vi "brc_daq_get_last_error.vi"(0 "return_value":i32) -> (19 "error out":errorcluster)   [LabVIEW 2019, in "BRC-DAQ.lvlib"]
uses:
  BRC-DAQ.lvlib
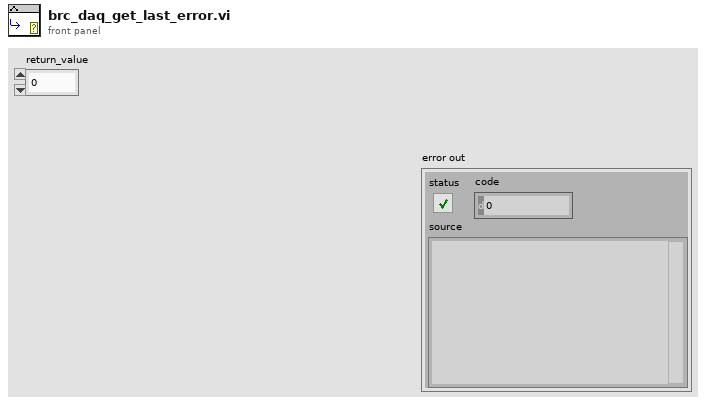
[diagram p1: front panel]
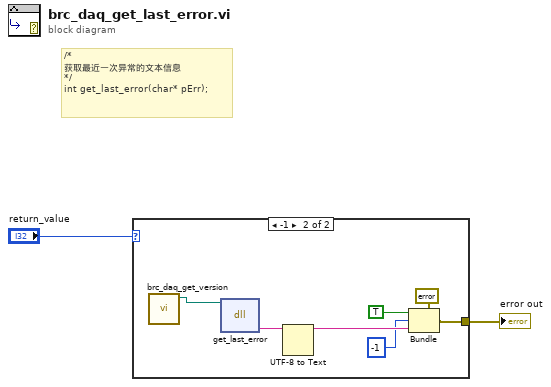
[diagram p0: block diagram]
diagram:
  # "/*\n获取最近一次异常的文本信息\n*/\nint get_last_error(char* pErr);"
  n1 = case shown="-1" "return_value" {
    tunnel: [_ w5] -> w2
    frame 0, Default {
    }
    frame -1 {
      n2 = call "brc_daq_get_version.vi"() -> ("dll path"=w3:path)  [unwired: 11 in]
      n3 = dll-call lib="E:/01 BRC project/04BRC-daq/04 Drive/DAQ-x64/DLL/brc_daq_sdk.dll" fn="get_last_error"(path in=w3) -> ("pErr"=w9:string)  [unwired: 4 in, 2 out]
      n4 = UTF-8 to Text(11:w9) -> (3:w7:string)  [unwired: 2 in, 1 out]
      n5 = Bundle(cluster=errorcluster {"status"=FALSE, "code"=0, "source"=""} ("error constant"), "status"=TRUE, "code"=-1, "source"=w7) -> (w5:errorcluster)
    }
  }
  "error out" <- w2
